vi "Initial States.vi"(8 "error in":errorcluster, 10 "States":string[](array[string]), 11 "Test Case In":refnum<class "Undo Redo Core.lvclass">) -> (0 "error out":errorcluster, 2 "Expected Undo Stack":string[](array[string]), 3 "Test Case Out":refnum<class "Undo Redo Core.lvclass">, 4 "Current State":string)   [LabVIEW 2021, in "Undo Redo Core.lvclass"]
uses:
  Undo Redo Core.lvclass
  C:/Program Files/National Instruments/LabVIEW 2024/vi.lib/Astemes/LUnit/Test Case.lvclass
  <resource>/plugins/NIIconEditor/Controls/Undo Redo Action.ctl
  <vilib>/Astemes/LUnit/Test Case.lvclass/Test Case.ctl
  48884588-6c28-42ca-a134-ce8f81f960ed.vi
  <vilib>/Astemes/LUnit/Append Pass Result.vi
  <vilib>/Astemes/LUnit/Append Fail Result.vi
  48884588-6c28-42ca-a134-ce8f81f960ed.vi/9c5d11cd-9439-4240-a1ee-d9baace9c924.vi
  <vilib>/Astemes/LUnit/Run In UI.vi
  <vilib>/Utility/error.llb/Clear Errors.vi
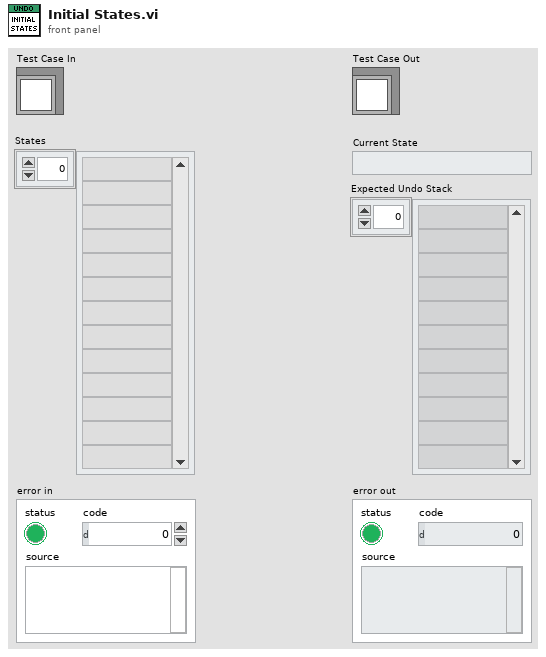
[diagram p1: front panel]
types:
  T1 = typedef "Undo Redo Action.ctl" = enum16{"Init", "Add", "Undo", "Redo", "Current State"}
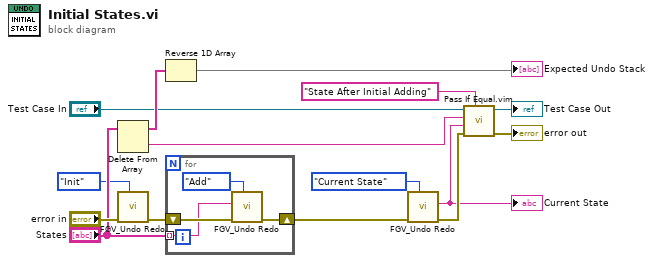
[diagram p0: block diagram]
diagram:
  n1 = Delete From Array(array="States") -> (deleted portion=w9:string, array with subset deleted=w15:string[])  [unwired: 2 in]
  n2 = call <resource>:"FGV_Undo Redo.vi"("Action"=Undo_Redo_Action."Init", "error in"="error in") -> ("error out"=w14:errorcluster)  [unwired: 7 in, 2 out]
  n3 = Reverse 1D Array(array=w15) -> (reversed array=→"Expected Undo Stack":string[])
  n4 = for {
    tunnel: "States" -> [w16] mode=indexing
    shift-right: [w18] -> w13
    shift-left: w14 -> [w19]
    n5 = call <resource>:"FGV_Undo Redo.vi"("Action"=Undo_Redo_Action."Add", "error in"=w19, "State In"=w16) -> ("error out"=w18:errorcluster)  [unwired: 6 in, 2 out]
  }
  n6 = call <resource>:"FGV_Undo Redo.vi"("Action"=Undo_Redo_Action."Current State", "error in"=w13) -> ("error out"=w12:errorcluster, "State Out"=w3:string)  [unwired: 7 in, 1 out]
  "Current State" <- w3
  n7 = call "Pass If Equal.vim"("Description"="State After Initial Adding", "error in (no error)"=w12, "Actual"=w3, "Expected"=w9, "LUnit Test Case In"="Test Case In") -> ("error out"=→"error out":errorcluster, "LUnit Test Case Out"=→"Test Case Out":refnum<class "Undo Redo Core.lvclass">)  [unwired: 5 in]
